vi "ziFlush.vi"(8 "error in":errorcluster, 11 "Handle In":T1 {"Handle" format="0x%08x"; "Conn" format="0x%08x"}) -> (0 "error out":errorcluster, 3 "Handle Out":T1 {"Handle" format="0x%08x"; "Conn" format="0x%08x"})   [LabVIEW 2018, in "Zurich Instruments LabOne.lvlib"]
doc: "Flush all data that currently is either in the server fifos or API fifos.\nTimeout is on 5 seconds."
uses:
  Zurich Instruments LabOne.lvlib
  ziTypeHandle.ctl
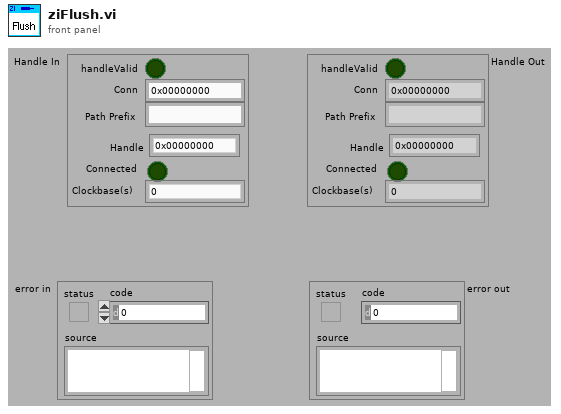
[diagram p1: front panel]
types:
  T1 = typedef "Zurich Instruments LabOne.lvlib/ziTypeHandle.ctl" = cluster{"handleValid":bool, "Conn":u64, "Path Prefix":string, "Handle":u64, "Connected":bool, "Clockbase(s)":dbl}
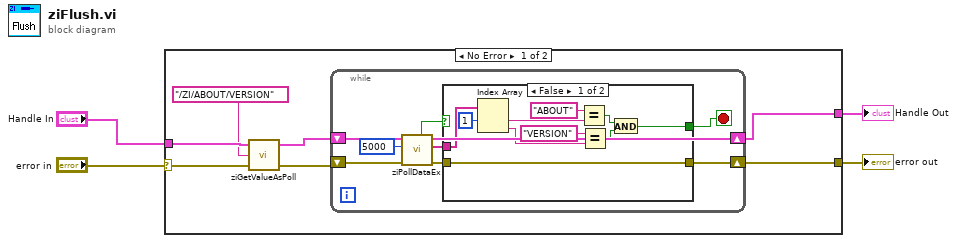
[diagram p0: block diagram]
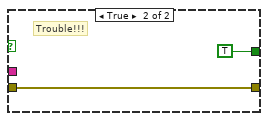
[diagram p2: hidden frame]
diagram:
  n1 = case shown="No Error" "error in" {
    selector: "error in" -> [w5 w33]
    tunnel: "Handle In" -> [w11 w34]
    tunnel: [w7 w34] -> w3
    tunnel: [w6 w33] -> w2
    frame No Error {
      n2 = call "ziGetValueAsPoll.vi"("error in"=w5, "Path"="/ZI/ABOUT/VERSION", "Handle in"=w11) -> ("error out"=w9:errorcluster, "Handle out"=w8:T1)  [unwired: 1 in]
      n3 = while {
        shift-right: [w13] -> w6
        shift-left: w9 -> [w19]
        shift-right: [w18] -> w7
        shift-left: w8 -> [w17]
        stop <- w14 stop-if-true
        n4 = call "ziPollDataEx.vi"("error in"=w19, "Timeout ms (50)"=5000 ("TimeOut ms (50)"), "Handle In"=w17) -> ("error out"=w12:errorcluster, "PathArray"=w16:string[], "Handle Out"=w18:T1, "Timed Out"=w15:bool)  [unwired: 1 in, 4 out]
        n5 = case shown="False" w15 {
          tunnel: w16 -> [w30 _]
          tunnel: [w22 TRUE] -> w14
          tunnel: [w21 w32] -> w13
          tunnel: w12 -> [w21 w32]
          frame False {
            n6 = Index Array(array=w30, index #1=1 ("index")) -> (element #1=w28:string, element #2=w25:string)  [unwired: 1 in]
            n7 = Equal?(x="ABOUT", y=w28) -> (x = y?=w23:bool)
            n8 = Equal?(x="VERSION", y=w25) -> (x = y?=w24:bool)
            n9 = And(x=w23, y=w24) -> (x .and. y?=w22:bool)
          }
          frame True {
            # "Trouble!!!"
          }
        }
      }
    }
    frame Error {
    }
  }
  "Handle Out" <- w3
  "error out" <- w2
